vi "Analiza_cazatura.vi"() -> ()   [LabVIEW 2018]
uses:
  <vilib>/Utility/file.llb/Read Delimited Spreadsheet (I64).vi
  <vilib>/Utility/file.llb/Write Delimited Spreadsheet (string).vi
  <vilib>/Utility/file.llb/Write Delimited Spreadsheet (I64).vi
panel:
  in  "Lungime pana la urmatorul prag":i32=50
  in  "Lungime fereastra":i32=100
  in  "Prag detectie":dbl=5.0 format="%#_13g"
  in  "ID_user":i32
  in  "Trial":i32=1
  out "Accel read":i64[](graph)
  out "Gyro read":i64[](graph)
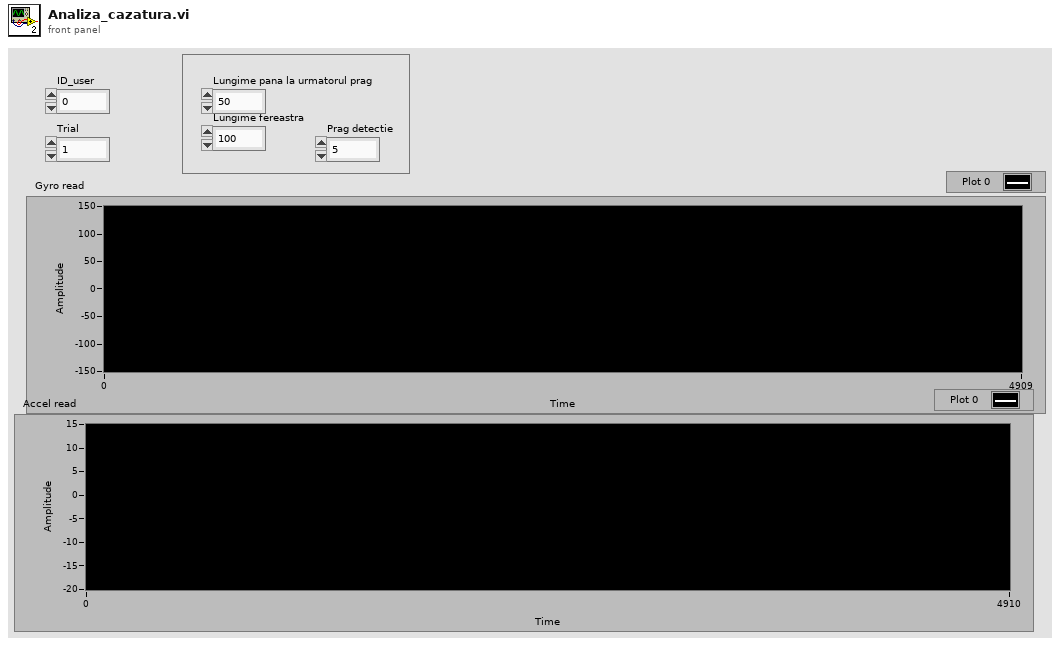
[diagram p1: front panel]
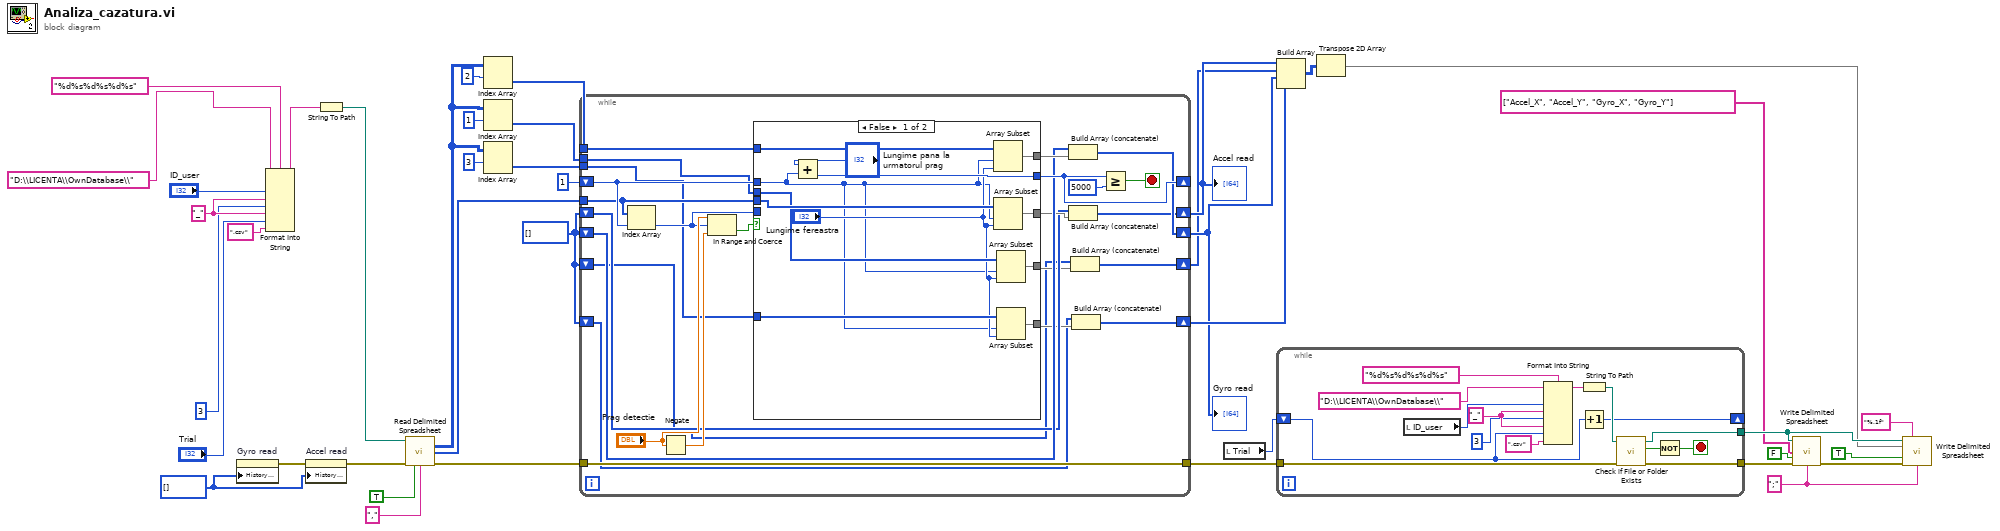
[diagram p0: block diagram]
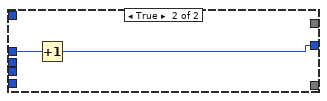
[diagram p2: hidden frame]
diagram:
  w26 = ";" ("delimiter (\\t)")
  w32 = "_"
  w13 = i64[] [] ("History Data")
  w5 = i64[] []
  n1 = property on="Gyro read" class="WFChart (strict)"("History Data"=w13) -> (error out=w12:errorcluster)  [unwired: 2 in, 1 out]
  n2 = Format Into String(format string="%d%s%d%s%d%s", initial string="D:\\LICENTA\\OwnDatabase\\", "ID_user", w32, 3 ("input 5"), w32, "Trial", ".csv" ("input 7")) -> (resulting string=w30:string)  [unwired: 1 in, 1 out]
  n3 = property on="Accel read" class="WFChart (strict)"(error in=w12, "History Data"=w13) -> (error out=w11:errorcluster)  [unwired: 1 in, 1 out]
  n4 = String To Path(string=w30) -> (path=w41:path)
  n5 = call-poly <vilib>:"Read Delimited Spreadsheet.vi"("file path (dialog if empty)"=w41, "error in (no error)"=w11, "transpose? (F)"=TRUE, "delimiter (\\t)"="," ("delimiter (\\t)")) -> ("all rows"=w8:i64[][], "first row"=w38:i64[], "error out"=w20:errorcluster)  [unwired: 6 in, 3 out]
  n6 = Index Array(array=w8, index (row)=2) -> (element=w35:i64[])  [unwired: 1 in]
  n7 = Index Array(array=w8, index (row)=1) -> (element=w7:i64[])  [unwired: 1 in]
  n8 = Index Array(array=w8, index (row)=3) -> (element=w6:i64[])  [unwired: 1 in]
  n9 = while {
    tunnel: w38 -> [w51]
    shift-right: [w61] -> _
    shift-left: 1 -> [w63]
    shift-right: [w58] -> w3
    shift-left: w5 -> [w56]
    tunnel: w35 -> [w52]
    shift-right: [w54] -> w16
    shift-left: w5 -> [w53]
    tunnel: w20 -> [w50]
    tunnel: [w50] -> w19
    tunnel: w7 -> [w49]
    tunnel: w6 -> [w48]
    shift-right: [w45] -> w4
    shift-left: w5 -> [w44]
    shift-right: [w43] -> w2
    shift-left: w5 -> [w42]
    stop <- w60 stop-if-true
    n10 = Index Array(array=w51, index=w63) -> (element=w62:i64)
    n11 = Negate(x="Prag detectie") -> (-x=w65:dbl)
    n12 = In Range and Coerce(upper limit="Prag detectie", x=w62, lower limit=w65) -> (In Range?=w64:bool)  [unwired: 1 out]
    n13 = case shown="False" w64 {
      tunnel: [w78 w79] -> w61
      tunnel: w63 -> [w69 w80]
      tunnel: w62 -> [_ _]
      tunnel: w52 -> [w77 _]
      tunnel: [w76 _] -> w57
      tunnel: w51 -> [w75 _]
      tunnel: [w74 _] -> w55
      tunnel: w49 -> [w72 _]
      tunnel: w48 -> [w71 _]
      tunnel: [w68 _] -> w47
      tunnel: [w67 _] -> w46
      frame False {
        n14 = Add(x="Lungime pana la urmatorul prag", y=w69) -> (x+y=w78:i32)
        n15 = Array Subset(array=w77, index=w69, length="Lungime fereastra") -> (w76:i64[])
        n16 = Array Subset(array=w75, index=w69, length="Lungime fereastra") -> (w74:i64[])
        n17 = Array Subset(array=w72, index=w69, length="Lungime fereastra") -> (w68:i64[])
        n18 = Array Subset(array=w71, index=w69, length="Lungime fereastra") -> (w67:i64[])
      }
      frame True {
        n19 = Increment(x=w80) -> (x+1=w79:i32)
      }
    }
    n20 = Build Array (concatenate)(w56, w57) -> (w58:i64[])
    n21 = Build Array (concatenate)(w53, w55) -> (w54:i64[])
    n22 = Build Array (concatenate)(w42, w47) -> (w43:i64[])
    n23 = Build Array (concatenate)(w44, w46) -> (w45:i64[])
    n24 = Greater Or Equal?(x=w61, y=5000) -> (x >= y?=w60:bool)
  }
  "Gyro read" <- w3
  "Accel read" <- w16
  n25 = local read "Trial"() -> (w21:i32)
  n26 = Build Array(w16, w2, w3, w4) -> (w15:i64[][])
  n27 = while {
    shift-right: [w92] -> _
    shift-left: w21 -> [w84]
    tunnel: [w91] -> w22
    tunnel: [w90] -> w24
    tunnel: w19 -> [w82]
    stop <- w93 stop-if-true
    w87 = "_"
    n28 = local read "ID_user"() -> (w83:i32)
    n29 = Format Into String(format string="%d%s%d%s%d%s", initial string="D:\\LICENTA\\OwnDatabase\\", w83, w87, 3 ("input 5"), w87, w84, ".csv" ("input 7")) -> (resulting string=w81:string)  [unwired: 1 in, 1 out]
    n30 = String To Path(string=w81) -> (path=w95:path)
    n31 = Increment(x=w84) -> (x+1=w92:i32)
    n32 = call <vilib>:"Check if File or Folder Exists.vi"("error in (no error)"=w82, "path"=w95) -> ("error out"=w91:errorcluster, "file or folder exists?"=w94:bool, "dup path"=w90:path)  [unwired: 7 in]
    n33 = Not(x=w94) -> (.not. x?=w93:bool)
  }
  n34 = Transpose 2D Array(2D array=w15) -> (transposed array=w14:i64[][])
  n35 = call-poly <vilib>:"Write Delimited Spreadsheet.vi"("file path (dialog if empty)"=w24, "1D data"=string[] ["Accel_X", "Accel_Y", "Gyro_X", "Gyro_Y"] ("Array"), "append to file? (new file:F)"=FALSE, "error in (no error)"=w22, "delimiter (\\t)"=w26) -> ("error out"=w23:errorcluster)  [unwired: 9 in, 1 out]
  n36 = call-poly <vilib>:"Write Delimited Spreadsheet.vi"("file path (dialog if empty)"=w24, "format (%d)"="%.1f" ("format (%.3f)"), "2D data"=w14, "append to file? (new file:F)"=TRUE, "error in (no error)"=w23, "delimiter (\\t)"=w26) -> ()  [unwired: 8 in, 2 out]
